vi "KE24xx, Read Current.vi"(7 "delay (100 ms)":dbl[unit]=0.1 format="%.1f", 8 "error in":errorcluster, 10 "Source Level (0.0 V)":dbl[unit] format="%.1f", 11 "VISA resource name":refnum<visa-resource-name>="GPIB0::9::INSTR") -> (0 "error out":errorcluster, 2 "Current":sgl[unit]=nan, 3 "VISA resource dup":refnum<visa-resource-name>)   [LabVIEW 2010]
uses:
  <instrlib>/Keithley 24XX/Keithley 24XX.lvlib
panel:
  in  "Number of Filter Readings (10)":u32=10
  in  "Filter Type  (1: Moving)":u16(ring)=1 items=["Repeating", "Moving"]
  in  "Enable Filter (T)":bool=TRUE
  in  "Mode (Triggered)":enum16{"IMM", "TRIGGERED"}(ring)=enum."TRIGGERED"
  in  "Source Function (volt)":enum16{"CURR", "VOLT"}(ring)=enum."VOLT"
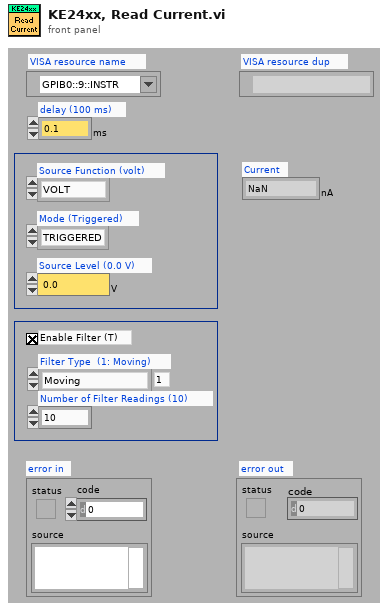
[diagram p1: front panel]
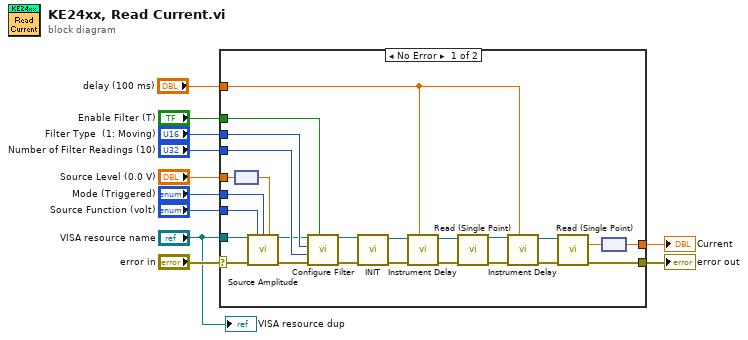
[diagram p0: block diagram]
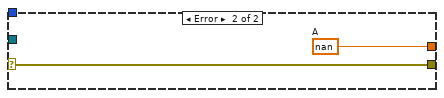
[diagram p2: hidden frame]
diagram:
  n1 = case shown="No Error" "error in" {
    selector: "error in" -> [w21 w38]
    tunnel: [w36 w37] -> w11
    tunnel: [w35 w38] -> w10
    tunnel: "Source Function (volt)" -> [w34 _]
    tunnel: "Mode (Triggered)" -> [w33 _]
    tunnel: "Source Level (0.0 V)" -> [w32 _]
    tunnel: "VISA resource name" -> [w31 _]
    tunnel: "Enable Filter (T)" -> [w30 _]
    tunnel: "Filter Type  (1: Moving)" -> [w29 _]
    tunnel: "Number of Filter Readings (10)" -> [w27 _]
    tunnel: "delay (100 ms)" -> [w15 _]
    frame No Error {
      n2 = node(w32) -> (w20:dbl)
      n3 = call "Source Amplitude.vi"("VISA resource name"=w31, "Source Function"=w34, "Mode"=w33, "Source Level"=w20, "error in (no error)"=w21) -> ("VISA resource name out"=w26:refnum<visa-resource-name>, "error out"=w28:errorcluster)  [unwired: 9 in]
      n4 = call <instrlib>:"Configure Filter.vi"("Enable Filter  (T: Enable)"=w30, "error in (no error)"=w28, "Number of Filter Readings (3)"=w27, "Filter Type  (0: Repeating)"=w29, "VISA resource name"=w26) -> ("error out"=w14:errorcluster, "VISA resource name out"=w13:refnum<visa-resource-name>)  [unwired: 5 in]
      n5 = call "INIT.vi"("VISA resource name"=w13, "error in (no error)"=w14) -> ("VISA resource name out"=w17:refnum<visa-resource-name>, "error out"=w19:errorcluster)  [unwired: 12 in]
      n6 = call "Instrument Delay.vi"("delay"=w15, "error in"=w19, "VISA resource"=w17) -> ("error out"=w18:errorcluster, "VISA resource dup"=w16:refnum<visa-resource-name>)  [unwired: 5 in]
      n7 = call <instrlib>:"Read (Single Point).vi"("VISA resource name"=w16, "error in (no error)"=w18) -> ("VISA resource name out"=w23:refnum<visa-resource-name>, "error out"=w24:errorcluster)  [unwired: 7 in, 5 out]
      n8 = call "Instrument Delay.vi"("delay"=w15, "error in"=w24, "VISA resource"=w23) -> ("error out"=w25:errorcluster, "VISA resource dup"=w22:refnum<visa-resource-name>)  [unwired: 5 in]
      n9 = call <instrlib>:"Read (Single Point).vi"("VISA resource name"=w22, "error in (no error)"=w25) -> ("Current"=w12:sgl, "error out"=w35:errorcluster)  [unwired: 7 in, 5 out]
      n10 = node(w12) -> (w36:sgl[unit])
    }
    frame Error {
      w37 = sgl[unit] nan  # A
    }
  }
  "Current" <- w11
  "error out" <- w10
  "VISA resource dup" <- "VISA resource name"
